vi "CB Discretize SSM.vi"(11 "Cont SSM":T2) -> (3 "State Space Model":T2)   [LabVIEW 2020]
uses:
  CB State Space.ctl
  <vilib>/Analysis/Matrix/Datatypes/RealMatrix.ctl
  <vilib>/Analysis/Matrix/Numeric/Conversions/Array To Matrix - RA2.vi
  <vilib>/Analysis/Matrix/Numeric/Multiply/Multiply - R,RM.vi
  <vilib>/Analysis/Matrix/Numeric/Exponential/Exponential - RM.vi
  <vilib>/Analysis/Matrix/NI_Matrix.lvlib
panel:
  out "e^A":T1
  out "Bd":T1
  out "Ad":T1
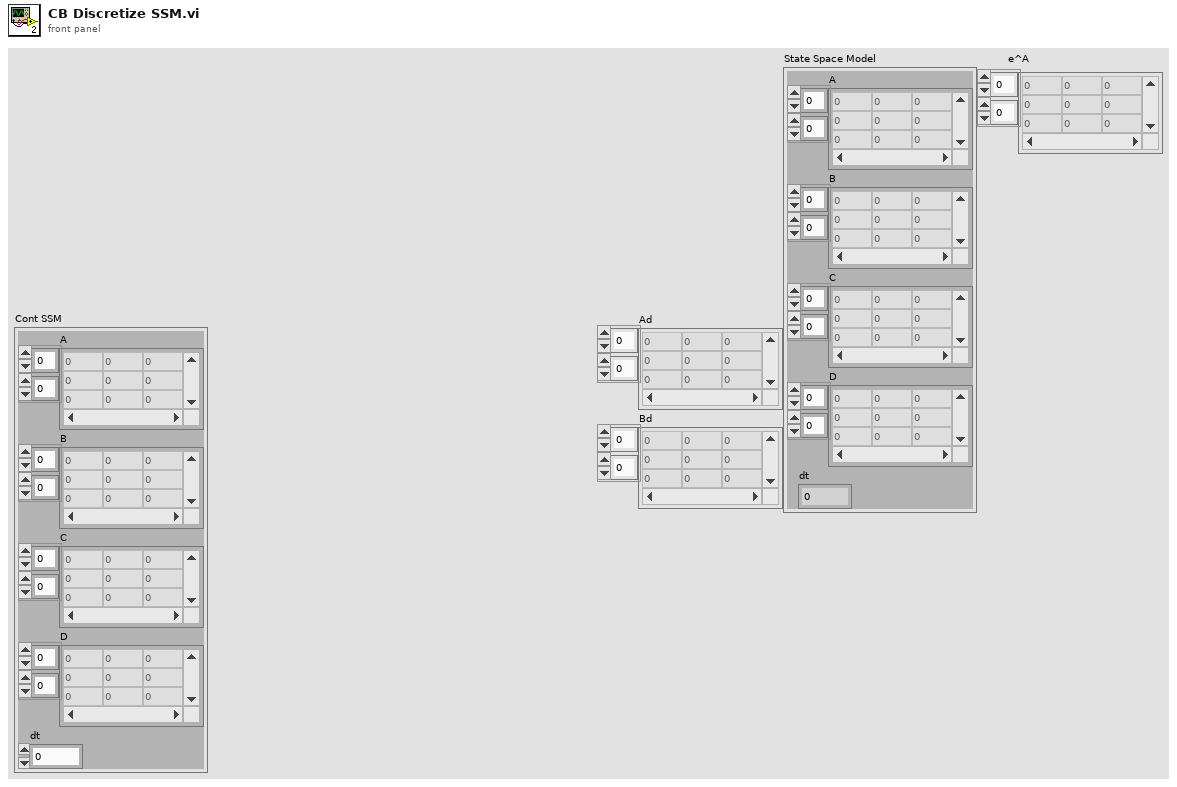
[diagram p1: front panel]
types:
  T1 = typedef "NI_Matrix.lvlib/RealMatrix.ctl" = dbl[][]
  T2 = typedef "CB State Space.ctl" = cluster{"A":T1, "B":T1, "C":T1, "D":T1, "dt":dbl}
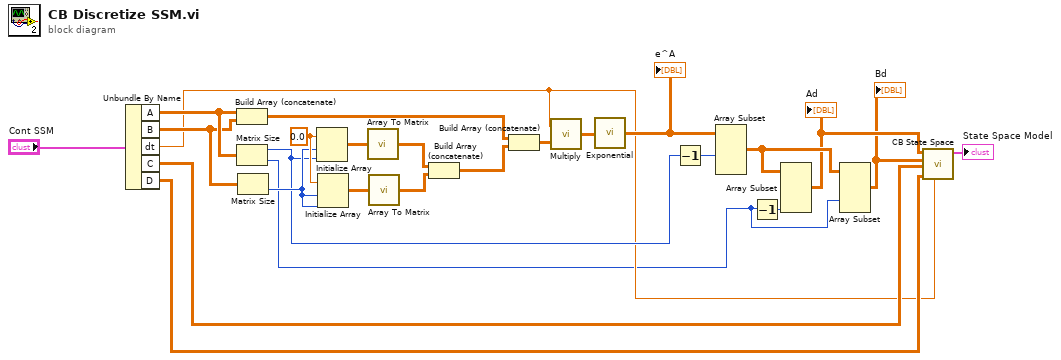
[diagram p0: block diagram]
diagram:
  w22 = 0.0 ("element")
  n1 = Unbundle By Name("Cont SSM") -> ("A"=w24:T1, "B"=w23:T1, "dt"=w4:dbl, "C"=w6:T1, "D"=w5:T1)
  n2 = Build Array (concatenate)(w24, w23) -> (w15:T1)
  n3 = Matrix Size(0:w24) -> (1:w11:i32, 2:w2:i32)
  n4 = Matrix Size(0:w23) -> (2:w21:i32)  [unwired: 1 out]
  n5 = Initialize Array(w22, w21, w11) -> (w20:dbl[][])
  n6 = Initialize Array(w22, w21, w21) -> (w19:dbl[][])
  n7 = call-poly <vilib>:"Array To Matrix.vi"("Real 2D Array"=w20) -> ("Real Matrix"=w18:T1)
  n8 = call-poly <vilib>:"Array To Matrix.vi"("Real 2D Array"=w19) -> ("Real Matrix"=w17:T1)
  n9 = Build Array (concatenate)(w18, w17) -> (w16:T1)
  n10 = Build Array (concatenate)(w15, w16) -> (w14:T1)
  n11 = call-poly <vilib>:"Multiply.vi"("Real Matrix A"=w14, "Real Scalar c"=w4) -> ("c * A"=w13:T1)
  n12 = call-poly <vilib>:"Exponential.vi"("Real Matrix A"=w13) -> ("e^A"=w12:T1)
  "e^A" <- w12
  n13 = Decrement(x=w11) -> (x-1=w10:i32)
  n14 = Array Subset(array=w12, length (row)=w10) -> (w9:T1)  [unwired: 3 in]
  n15 = Decrement(x=w2) -> (x-1=w1:i32)
  n16 = Array Subset(array=w9, length (col)=w1) -> (w8:T1)  [unwired: 3 in]
  "Ad" <- w8
  n17 = Array Subset(array=w9, index (col)=w2) -> (w7:T1)  [unwired: 3 in]
  "Bd" <- w7
  n18 = call "CB State Space.vi"("dt"=w4, "D"=w5, "C"=w6, "B"=w7, "A"=w8) -> ("State Space Model"=→"State Space Model":T2)  [unwired: 5 in, 1 out]
